vi "Check For Duplicate Unique Names.vi"(8 "error in (no error)":errorcluster, 11 "VI Panel Layout in":refnum<class "VI Panel Layout.lvclass">) -> (0 "error out":errorcluster, 1 "duplicate names":string[](array[string]), 2 "duplicates found?":bool, 3 "VI Panel Layout out":refnum<class "VI Panel Layout.lvclass">)   [LabVIEW 2012, in "NI_SE_Front Panel Layout.lvlib" / "VI Panel Layout.lvclass"]
doc: "Check if any of the object layouts have duplicate unique names."
uses:
  VI Panel Layout.lvclass
  VI Panel Layout.lvclass/VI Panel Layout.ctl
  Object Layout Classes/Object Layout/Object Layout.lvclass/Object Layout.ctl
  Object Layout Classes/Object Layout/Object Layout.lvclass
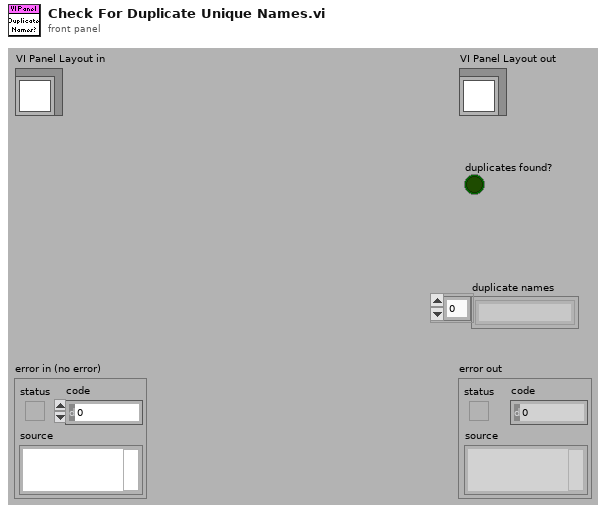
[diagram p1: front panel]
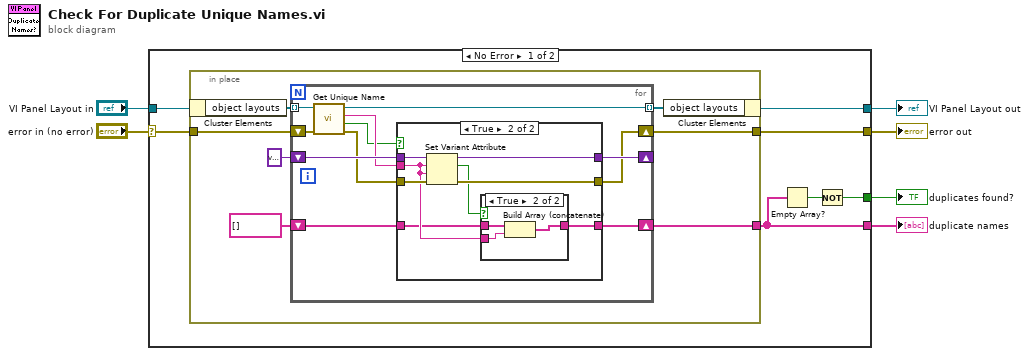
[diagram p0: block diagram]
diagram:
  n1 = case shown="No Error" "error in (no error)" {
    selector: "error in (no error)" -> [w11 w48]
    tunnel: [w10 w48] -> w5
    tunnel: [w12 w47] -> w3
    tunnel: "VI Panel Layout in" -> [w13 w47]
    tunnel: [w8 _] -> w2
    tunnel: [w7 _] -> w1
    frame No Error {
      n2 = in-place {
        in-place-border: w11 -> [w18]
        in-place-border: [w17] -> w10
        in-place-border: [w14] -> w7
        n3 = in-place-cluster #1(w13) -> ("object layouts"=w20:refnum<class "Object Layout.lvclass">[])
        n4 = for {
          tunnel: w20 -> [w31] mode=indexing
          tunnel: [w30] -> w19 mode=indexing
          shift-right: [w23] -> w17
          shift-left: w18 -> [w29]
          shift-right: [w28] -> _
          shift-left: variant -> [w27]
          shift-right: [w22] -> w14
          shift-left: string[] [] -> [w21]
          n5 = call "Get Unique Name.vi"("error in (no error)"=w29, "Object Layout in"=w31) -> ("error out"=w25:errorcluster, "found?"=w24:bool, "unique name"=w26:string, "Object Layout out"=w30:refnum<class "Object Layout.lvclass">)  [unwired: 6 in]
          n6 = case shown="True" w24 {
            tunnel: [w34 w42] -> w28
            tunnel: w27 -> [w34 w41]
            tunnel: w26 -> [_ w37]
            tunnel: w25 -> [w33 w40]
            tunnel: [w33 w39] -> w23
            tunnel: [w32 w36] -> w22
            tunnel: w21 -> [w32 w35]
            frame False {
            }
            frame True {
              n7 = Set Variant Attribute(Variant=w41, name=w37, value=w37, error in=w40) -> (Variant out=w42:variant, replaced=w38:bool, error out=w39:errorcluster)
              n8 = case shown="True" w38 {
                tunnel: w37 -> [_ w46]
                tunnel: [w43 w45] -> w36
                tunnel: w35 -> [w43 w44]
                frame False {
                }
                frame True {
                  n9 = Build Array (concatenate)(w44, w46) -> (w45:string[])
                }
              }
            }
          }
        }
        n10 = in-place-cluster #1("object layouts"=w19) -> (w12:refnum<class "VI Panel Layout.lvclass">)
      }
      n11 = Empty Array?(array=w7) -> (empty?=w9:bool)
      n12 = Not(x=w9) -> (.not. x?=w8:bool)
    }
    frame Error {
    }
  }
  "error out" <- w5
  "VI Panel Layout out" <- w3
  "duplicates found?" <- w2
  "duplicate names" <- w1
